vi "WLAN - TV - RW - UTIL - TestVectors_11AC.vi"(0 "TV_IQComposite_11N":T2={"Standard"=3, "FEC Coding Type"=[0], "Guard Interval (s)"=[0.0], "OFDM Advanced Controls"={"OFDM Auto Compute Acquisition Length Enabled"=0, "OFDM Maximum Symbols Used"=0, "OFDM Time Tracking Enabled"=0, "OFDM Channel Tracking Enabled"=0, "OFDM Amplitude Tracking Enabled"=1, "OFDM CFO Estimation Method"=0, "OFDM Phase Tracking Method"=0, "OFDM Header Detection Enabled"=0, "OFDM MAC FCS Check Enabled"=0, "#Avg"=10, "#Iterations"=10}, "Generation Parameters"=[], "Measurement Enabled"=TRUE, "#Packets"=0} {"Generation Parameters"."Center Frequency(Hz)" format="%#_6p"; "Generation Parameters"."Generation Parameters"."Channel BW(Hz)" items=["5M"=5000000.0, "10M"=10000000.0, "20M"=20000000.0, "40M"=40000000.0, "80M"=80000000.0, "160M"=160000000.0]; "OFDM Advanced Controls"."OFDM Phase Tracking Method" items=["Standard", "Instantaneous", "None", "Standard with Cubic Spline Fit"]; "OFDM Advanced Controls"."OFDM CFO Estimation Method" items=["Preamble Only", "Preamble and Data"]; "OFDM Advanced Controls"."OFDM Channel Tracking Enabled" items=["False", "True"]; "OFDM Advanced Controls"."OFDM Amplitude Tracking Enabled" items=["False", "True"]; "OFDM Advanced Controls"."OFDM Time Tracking Enabled" items=["True"=1, "False"=0]; "OFDM Advanced Controls"."OFDM Auto Compute Acquisition Length Enabled" items=["False", "True"]; "OFDM Advanced Controls"."OFDM MAC FCS Check Enabled" items=["False", "True"]; "OFDM Advanced Controls"."OFDM Header Detection Enabled" items=["False", "True"]; "FEC Coding Type" items=["BCC", "LDPC"]; "Standard" items=["80211A/G/J/P OFDM", "80211B/G DSSS", "80211G DSSSOFDM", "80211N MIMOOFDM", "80211AC MIMOOFDM"]}, 1 "11ac_Meas_Config":path, 3 "TV_802_11ac":path, 9 "TV Paramaters":T1) -> ()   [LabVIEW 2011]
uses:
  Includes/WLAN - TV - RW - INC - TV_IQComposite_11AC.ctl
  Includes/WLAN - TV - RW - INC - TV_OFDM Demod.ctl
  Includes/WLAN - TV - RW - INC - TV_Parameters.ctl
  Includes/WLAN - TV - RW - INC - Tx_Meas_Settings_OFDM_String.ctl
  <vilib>/Utility/file.llb/Write To Spreadsheet File (string).vi
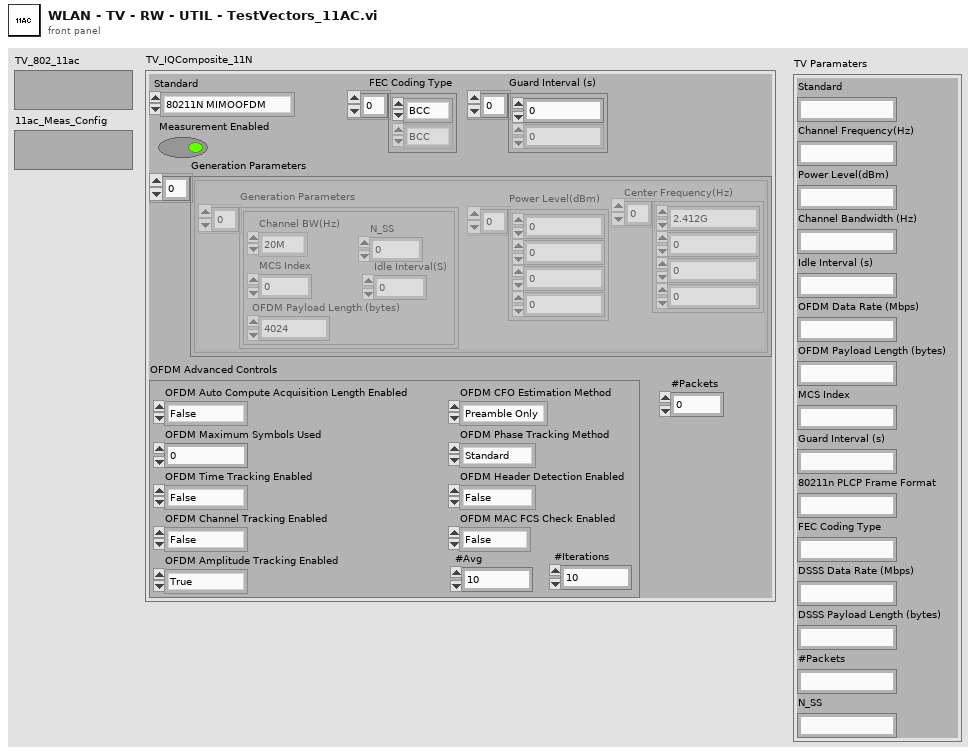
[diagram p1: front panel]
types:
  T1 = typedef "WLAN - TV - RW - INC - TV_Parameters.ctl" = cluster{"Standard ":string, "Channel Frequency(Hz)":string, "Power Level(dBm)":string, "Channel Bandwidth (Hz)":string, "Idle Interval (s)":string, "OFDM Data Rate (Mbps)":string, "OFDM Payload Length (bytes)":string, "MCS Index":string, "Guard Interval (s)":string, "80211n PLCP Frame Format":string, "FEC Coding Type":string, "DSSS Data Rate (Mbps)":string, "DSSS Payload Length (bytes)":string, "#Packets":string, "N_SS":string}
  T2 = typedef "WLAN - TV - RW - INC - TV_IQComposite_11AC.ctl" = cluster{"Standard":i32, "FEC Coding Type":i32[], "Guard Interval (s)":dbl[], "OFDM Advanced Controls":T3, "Generation Parameters":cluster{"Generation Parameters":cluster{"Channel BW(Hz)":dbl, "MCS Index":i32, "OFDM Payload Length (bytes)":i32, "Idle Interval(S)":dbl, "N_SS":i32}[], "Center Frequency(Hz)":dbl[], "Power Level(dBm)":dbl[]}[], "Measurement Enabled":bool, "#Packets":i32}
  T3 = typedef "WLAN - TV - RW - INC - TV_OFDM Demod.ctl" = cluster{"OFDM Auto Compute Acquisition Length Enabled":i32, "OFDM Maximum Symbols Used":i32, "OFDM Time Tracking Enabled":i32, "OFDM Channel Tracking Enabled":i32, "OFDM Amplitude Tracking Enabled":i32, "OFDM CFO Estimation Method":i32, "OFDM Phase Tracking Method":i32, "OFDM Header Detection Enabled":i32, "OFDM MAC FCS Check Enabled":i32, "#Avg":i32, "#Iterations":i32}
  T4 = typedef "WLAN - TV - RW - INC - Tx_Meas_Settings_OFDM_String.ctl" = cluster{"OFDM Auto Compute Acquisition Length Enabled":string, "OFDM Maximum Symbols Used":string, "OFDM Time Tracking Enabled":string, "OFDM Channel Tracking Enabled":string, "OFDM Amplitude Tracking Enabled":string, "OFDM CFO Estimation Method":string, "OFDM Phase Tracking Method":string, "OFDM Header Detection Enabled":string, "OFDM MAC FCS Check Enabled":string, "#Avg":string, "#Iterations":string}
  T5 = cluster{"Generation Parameters":cluster{"Channel BW(Hz)":dbl, "MCS Index":i32, "OFDM Payload Length (bytes)":i32, "Idle Interval(S)":dbl, "N_SS":i32}[], "Center Frequency(Hz)":dbl[], "Power Level(dBm)":dbl[]}[]
  T6 = cluster{"Channel BW(Hz)":dbl, "MCS Index":i32, "OFDM Payload Length (bytes)":i32, "Idle Interval(S)":dbl, "N_SS":i32}[]
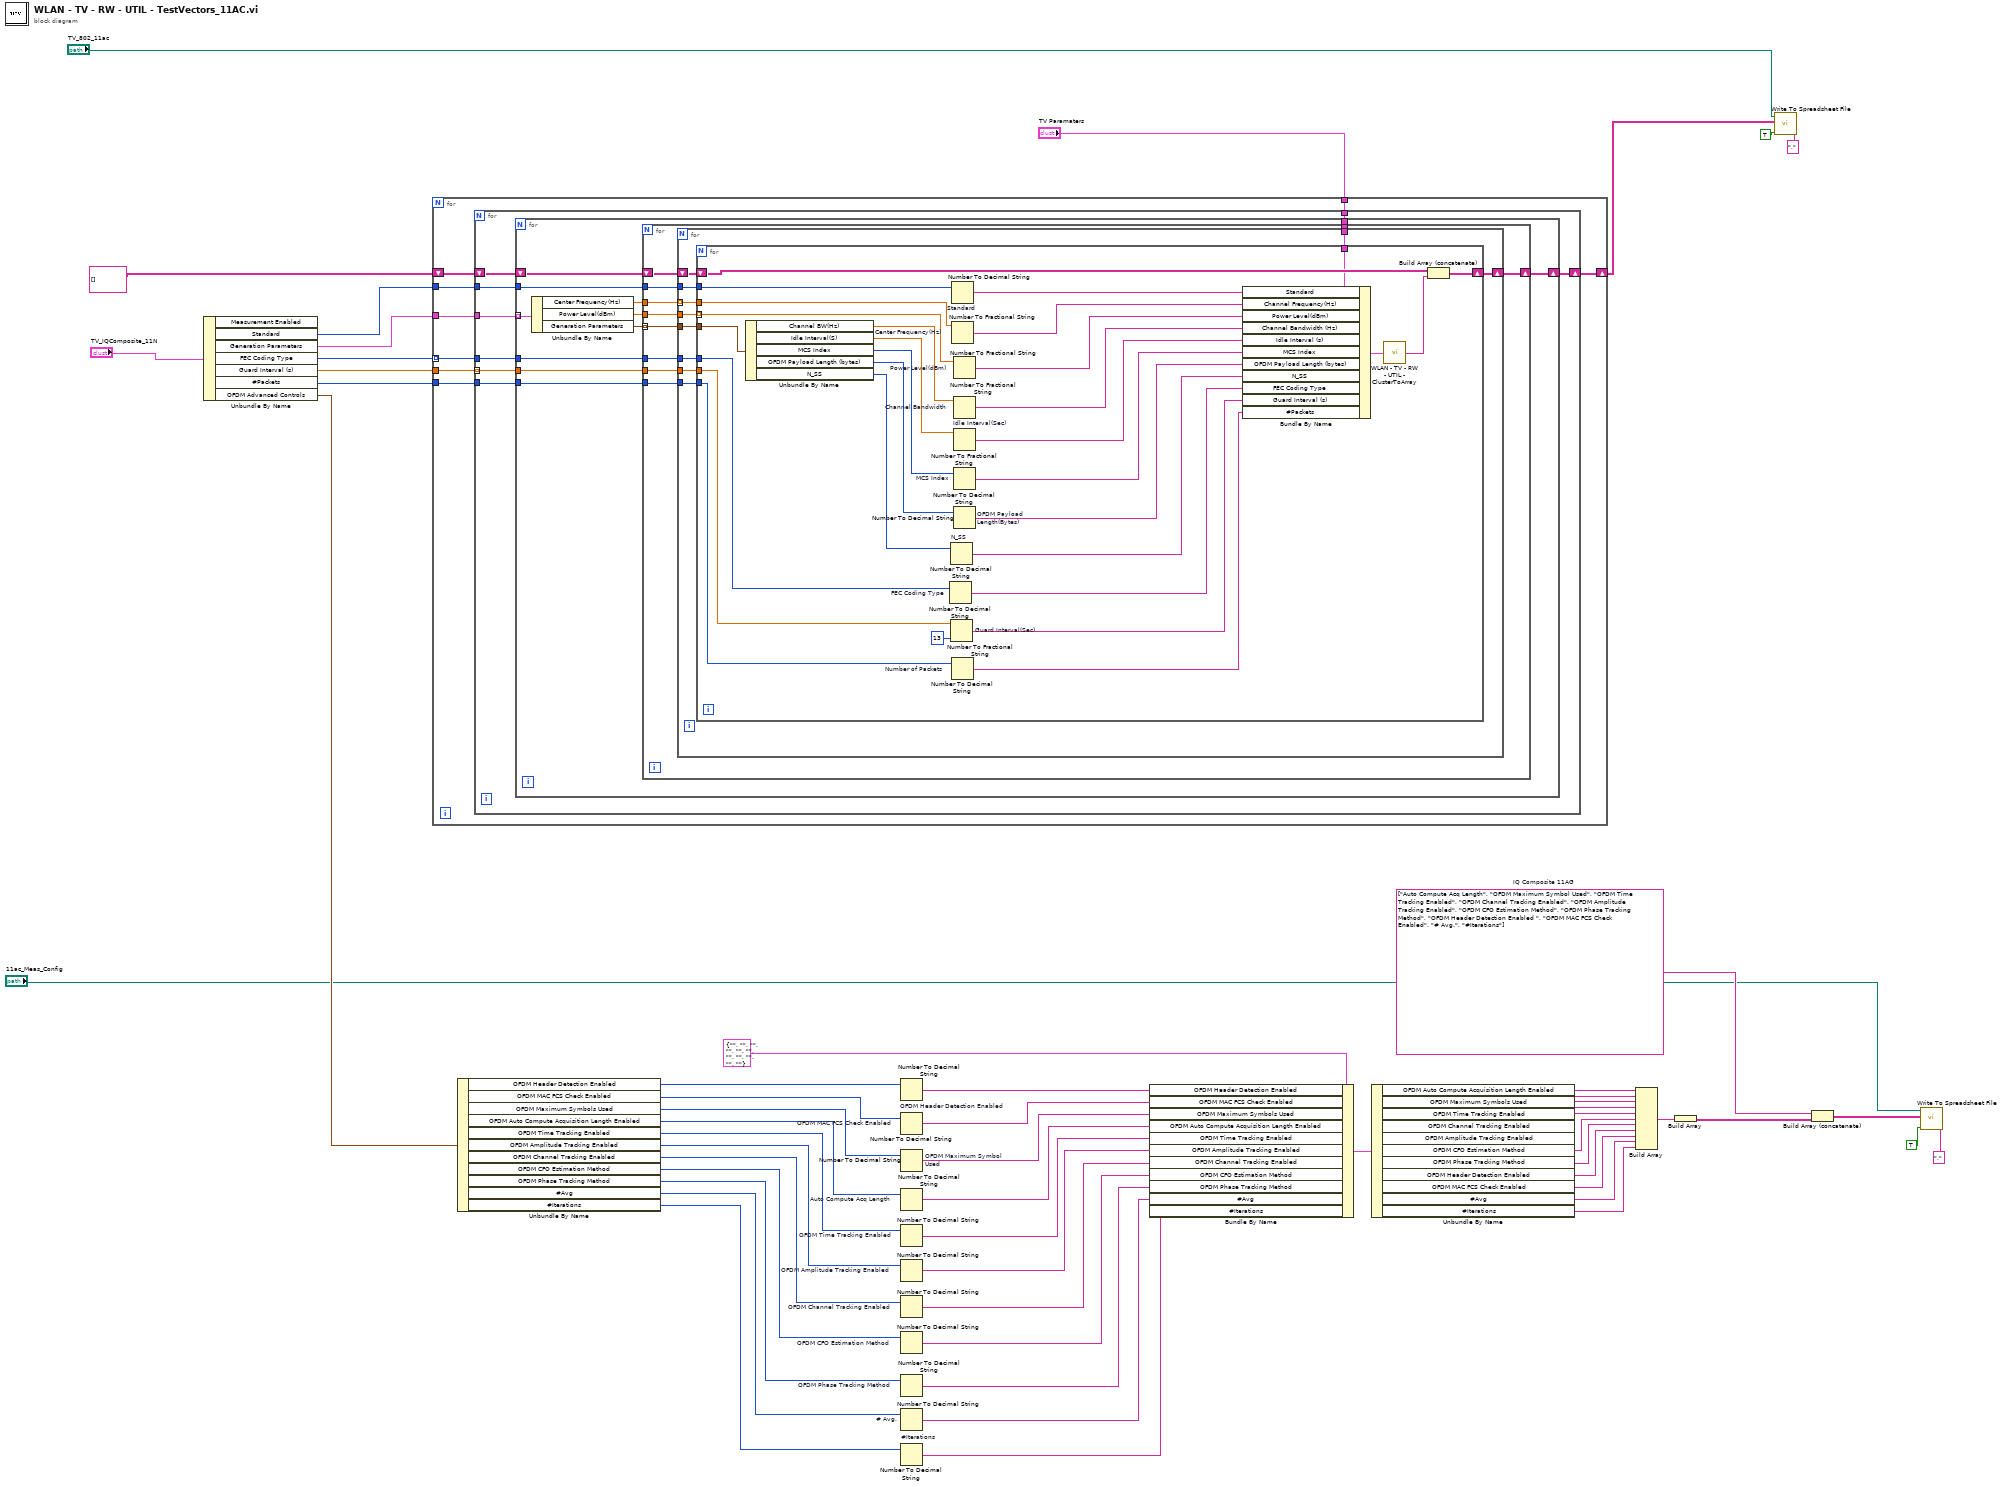
[diagram p0: block diagram]
diagram:
  w7 = string[] ["Auto Compute Acq Length", "OFDM Maximum Symbol Used", "OFDM Time Tracking Enabled", "OFDM Channel Tracking Enabled", "OFDM Amplitude Tracking Enabled", "OFDM CFO Estimation Method", "OFDM Phase Tracking Method", "OFDM Header Detection Enabled ", "OFDM MAC FCS Check Enabled", "# Avg.", "#Iterations"]  # IQ Composite 11AG
  n1 = Unbundle By Name("TV_IQComposite_11N") -> ("Standard"=w51:i32, "Generation Parameters"=w47:T5, "FEC Coding Type"=w55:i32[], "Guard Interval (s)"=w54:dbl[], "#Packets"=w46:i32, "OFDM Advanced Controls"=w4:T3)  [unwired: 1 out]
  n2 = for {
    tunnel: w55 -> [w63] mode=indexing
    tunnel: w54 -> [w62]
    tunnel: w51 -> [w61]
    tunnel: "TV Paramaters" -> [w60]
    shift-right: [w59] -> w1
    shift-left: string[][] [] ("appended array") -> [w58]
    tunnel: w47 -> [w57]
    tunnel: w46 -> [w56]
    n3 = for {
      tunnel: w63 -> [w71]
      tunnel: w62 -> [w70] mode=indexing
      tunnel: w61 -> [w69]
      tunnel: w60 -> [w68]
      shift-right: [w67] -> w59
      shift-left: w58 -> [w66]
      tunnel: w57 -> [w65]
      tunnel: w56 -> [w64]
      n4 = for {
        tunnel: w71 -> [w74]
        tunnel: w70 -> [w73]
        tunnel: w69 -> [w82]
        tunnel: w68 -> [w81]
        shift-right: [w80] -> w67
        shift-left: w66 -> [w76]
        tunnel: w65 -> [w75] mode=indexing
        tunnel: w64 -> [w72]
        n5 = Unbundle By Name(w75) -> ("Center Frequency(Hz)"=w78:dbl[], "Power Level(dBm)"=w77:dbl[], "Generation Parameters"=w79:T6)
        n6 = for {
          tunnel: w82 -> [w92]
          tunnel: w81 -> [w91]
          tunnel: w79 -> [w89] mode=indexing
          tunnel: w78 -> [w88]
          tunnel: w77 -> [w87]
          shift-right: [w90] -> w80
          shift-left: w76 -> [w86]
          tunnel: w74 -> [w85]
          tunnel: w73 -> [w84]
          tunnel: w72 -> [w83]
          n7 = for {
            shift-right: [w101] -> w90
            shift-left: w86 -> [w102]
            tunnel: w92 -> [w100]
            tunnel: w91 -> [w99]
            tunnel: w89 -> [w98]
            tunnel: w88 -> [w97] mode=indexing
            tunnel: w87 -> [w96]
            tunnel: w85 -> [w95]
            tunnel: w84 -> [w94]
            tunnel: w83 -> [w93]
            n8 = for {
              shift-right: [w131] -> w101
              shift-left: w102 -> [w130]
              tunnel: w100 -> [w129]
              tunnel: w99 -> [w127]
              tunnel: w98 -> [w114]
              tunnel: w97 -> [w115]
              tunnel: w96 -> [w116] mode=indexing
              tunnel: w95 -> [w109]
              tunnel: w94 -> [w108]
              tunnel: w93 -> [w107]
              n9 = Unbundle By Name(w114) -> ("Channel BW(Hz)"=w110:dbl, "Idle Interval(S)"=w111:dbl, "MCS Index"=w112:i32, "OFDM Payload Length (bytes)"=w113:i32, "N_SS"=w103:i32)
              n10 = Number To Decimal String "FEC Coding Type"(number=w109) -> (decimal integer string=w117:string)  [unwired: 1 in]
              n11 = Number To Decimal String "N_SS"(number=w103) -> (decimal integer string=w104:string)  [unwired: 1 in]
              n12 = Number To Fractional String "Guard Interval(Sec)"(number=w108, precision (6)=i16 13) -> (F-format string=w118:string)  [unwired: 2 in]
              n13 = Number To Decimal String "Number of Packets"(number=w107) -> (decimal integer string=w106:string)  [unwired: 1 in]
              n14 = Number To Decimal String "Standard"(number=w129) -> (decimal integer string=w119:string)  [unwired: 1 in]
              n15 = Number To Fractional String "Center Frequency(Hz)"(number=w115) -> (F-format string=w120:string)  [unwired: 3 in]
              n16 = Number To Fractional String "Power Level(dBm)"(number=w116) -> (F-format string=w121:string)  [unwired: 3 in]
              n17 = Number To Fractional String "Channel Bandwidth"(number=w110) -> (F-format string=w122:string)  [unwired: 3 in]
              n18 = Number To Fractional String "Idle Interval(Sec)"(number=w111) -> (F-format string=w123:string)  [unwired: 3 in]
              n19 = Number To Decimal String "MCS Index"(number=w112) -> (decimal integer string=w124:string)  [unwired: 1 in]
              n20 = Number To Decimal String "OFDM Payload Length(Bytes)"(number=w113) -> (decimal integer string=w125:string)  [unwired: 1 in]
              n21 = Bundle By Name(cluster=w127, "Standard"=w119, "Channel Frequency(Hz)"=w120, "Power Level(dBm)"=w121, "Channel Bandwidth (Hz)"=w122, "Idle Interval (s)"=w123, "MCS Index"=w124, "OFDM Payload Length (bytes)"=w125, "N_SS"=w104, "FEC Coding Type"=w117, "Guard Interval (s)"=w118, "#Packets"=w106) -> (w126:T1)
              n22 = call "WLAN - TV - RW - UTIL - ClusterToArray.vi"("TV Paramaters"=w126) -> ("TV_Parameters(1-D array)"=w128:string[])  [unwired: 14 in]
              n23 = Build Array (concatenate)(w130, w128) -> (w131:string[][])
            }
          }
        }
      }
    }
  }
  n24 = Unbundle By Name(w4) -> ("OFDM Header Detection Enabled"=w35:i32, "OFDM MAC FCS Check Enabled"=w36:i32, "OFDM Maximum Symbols Used"=w37:i32, "OFDM Auto Compute Acquisition Length Enabled"=w38:i32, "OFDM Time Tracking Enabled"=w39:i32, "OFDM Amplitude Tracking Enabled"=w40:i32, "OFDM Channel Tracking Enabled"=w41:i32, "OFDM CFO Estimation Method"=w42:i32, "OFDM Phase Tracking Method"=w43:i32, "#Avg"=w44:i32, "#Iterations"=w45:i32)
  n25 = Number To Decimal String "OFDM Header Detection Enabled"(number=w35) -> (decimal integer string=w33:string)  [unwired: 1 in]
  n26 = Number To Decimal String "OFDM MAC FCS Check Enabled"(number=w36) -> (decimal integer string=w32:string)  [unwired: 1 in]
  n27 = Number To Decimal String "OFDM Maximum Symbol Used"(number=w37) -> (decimal integer string=w31:string)  [unwired: 1 in]
  n28 = Number To Decimal String "Auto Compute Acq Length"(number=w38) -> (decimal integer string=w30:string)  [unwired: 1 in]
  n29 = Number To Decimal String "OFDM Time Tracking Enabled"(number=w39) -> (decimal integer string=w29:string)  [unwired: 1 in]
  n30 = Number To Decimal String "OFDM Amplitude Tracking Enabled"(number=w40) -> (decimal integer string=w28:string)  [unwired: 1 in]
  n31 = Number To Decimal String "OFDM Channel Tracking Enabled"(number=w41) -> (decimal integer string=w23:string)  [unwired: 1 in]
  n32 = Number To Decimal String "OFDM CFO Estimation Method"(number=w42) -> (decimal integer string=w24:string)  [unwired: 1 in]
  n33 = Number To Decimal String "OFDM Phase Tracking Method"(number=w43) -> (decimal integer string=w25:string)  [unwired: 1 in]
  n34 = Number To Decimal String "# Avg."(number=w44) -> (decimal integer string=w26:string)  [unwired: 1 in]
  n35 = Number To Decimal String "#Iterations"(number=w45) -> (decimal integer string=w27:string)  [unwired: 1 in]
  n36 = Bundle By Name(cluster=T4 {"OFDM Auto Compute Acquisition Length Enabled"="", "OFDM Maximum Symbols Used"="", "OFDM Time Tracking Enabled"="", "OFDM Channel Tracking Enabled"="", "OFDM Amplitude Tracking Enabled"="", "OFDM CFO Estimation Method"="", "OFDM Phase Tracking Method"="", "OFDM Header Detection Enabled"="", "OFDM MAC FCS Check Enabled"="", "#Avg"="", "#Iterations"=""} ("OFDM Measurement Settings"), "OFDM Header Detection Enabled"=w33, "OFDM MAC FCS Check Enabled"=w32, "OFDM Maximum Symbols Used"=w31, "OFDM Auto Compute Acquisition Length Enabled"=w30, "OFDM Time Tracking Enabled"=w29, "OFDM Amplitude Tracking Enabled"=w28, "OFDM Channel Tracking Enabled"=w23, "OFDM CFO Estimation Method"=w24, "OFDM Phase Tracking Method"=w25, "#Avg"=w26, "#Iterations"=w27) -> (w20:T4)
  n37 = Unbundle By Name(w20) -> ("OFDM Auto Compute Acquisition Length Enabled"=w19:string, "OFDM Maximum Symbols Used"=w18:string, "OFDM Time Tracking Enabled"=w17:string, "OFDM Channel Tracking Enabled"=w16:string, "OFDM Amplitude Tracking Enabled"=w15:string, "OFDM CFO Estimation Method"=w14:string, "OFDM Phase Tracking Method"=w13:string, "OFDM Header Detection Enabled"=w12:string, "OFDM MAC FCS Check Enabled"=w11:string, "#Avg"=w10:string, "#Iterations"=w9:string)
  n38 = Build Array(w19, w18, w17, w16, w15, w14, w13, w12, w11, w10, w9) -> (w8:string[])
  n39 = Build Array(w8) -> (w5:string[][])
  n40 = call-poly <vilib>:"Write To Spreadsheet File.vi"("delimiter (\\t)"="," ("delimiter (\\t)"), "append to file? (new file:F)"=TRUE, "2D data"=w1, "file path (dialog if empty)"="TV_802_11ac") -> ()  [unwired: 4 in, 1 out]
  n41 = Build Array (concatenate)(w7, w5) -> (w6:string[][])
  n42 = call-poly <vilib>:"Write To Spreadsheet File.vi"("delimiter (\\t)"="," ("delimiter (\\t)"), "append to file? (new file:F)"=TRUE, "2D data"=w6, "file path (dialog if empty)"="11ac_Meas_Config") -> ()  [unwired: 4 in, 1 out]
